vi "DAC Configure.vi"(8 "error in":errorcluster, 11 "DAC DC Supply in":refnum<class "DAC DC Supply.lvclass">) -> (0 "error out":errorcluster, 3 "DAC DC Supply out":refnum<class "DAC DC Supply.lvclass">)   [LabVIEW 2019, in "DAC.lvlib" / "DAC DC Supply.lvclass"]
uses:
  DAC DC Supply.lvclass
  C:/Users/krio/Documents/LV_Projects/test-stand/App/DAC/DAC.lvclass
  DAC.lvclass/DAC.ctl
  DAC DC Supply.lvclass/DAC DC Supply.ctl
  DAC.lvclass
  <instrlib>/Agilent 66XX Series/Agilent 66XX Series.lvlib
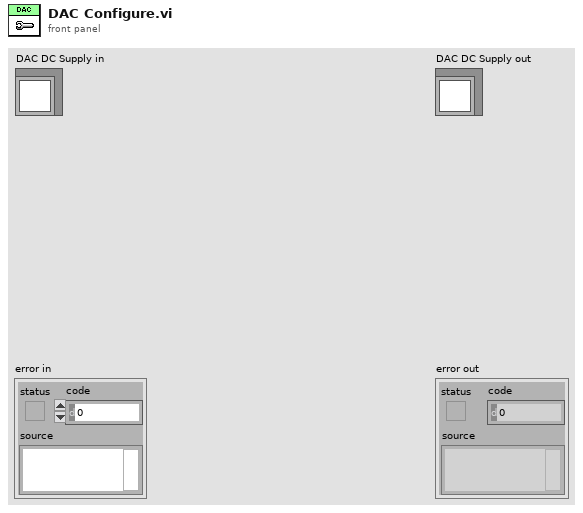
[diagram p1: front panel]
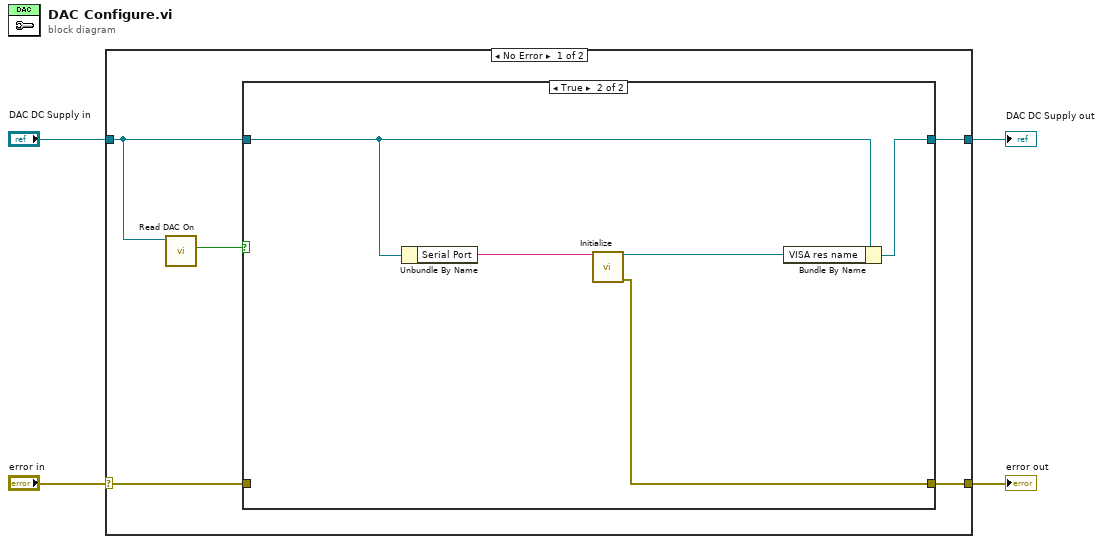
[diagram p0: block diagram]
diagram:
  n1 = case shown="No Error" "error in" {
    selector: "error in" -> [w6 w18]
    tunnel: [w5 w18] -> w4
    tunnel: [w7 w17] -> w3
    tunnel: "DAC DC Supply in" -> [w9 w17]
    frame No Error {
      n2 = call "Read DAC On.vi"("DAC in"=w9) -> ("DAC On"=w8:bool)  [unwired: 8 in, 2 out]
      n3 = case shown="True" w8 {
        tunnel: w9 -> [w11 w16]
        tunnel: [w11 w15] -> w7
        tunnel: w6 -> [w10 _]
        tunnel: [w10 w12] -> w5
        frame False {
          # "Temperature measurement is off."
        }
        frame True {
          # "Temperature measurement is on."
          n4 = Unbundle By Name(w16) -> ("Serial Port"=w14:string)
          n5 = call <instrlib>:"Initialize.vi"("VISA resource name"=w14) -> ("VISA resource name out"=w13:refnum<visa-resource-name>, "error out"=w12:errorcluster)  [unwired: 13 in]
          n6 = Bundle By Name(cluster=w16, "VISA res name"=w13) -> (w15:refnum<class "DAC DC Supply.lvclass">)
        }
      }
    }
    frame Error {
    }
  }
  "error out" <- w4
  "DAC DC Supply out" <- w3
